vi "LcWebView_AlertDialog_Example2.vi"() -> ()   [LabVIEW 2018, in "LcWebView.lvclass"]
doc: "Inject javascript arguments"
uses:
  LcWebView.lvclass
  C:/Projects/LcWebView2/LcWebView/LcWebView_class/data/Microsoft.Web.WebView2.WinForms.dll
  data/Microsoft.Web.WebView2.WinForms.dll
panel:
  out "BrowserProcessId":u32
  out "Status Message":string
  in  "stop":bool
  in  "Web":refnum<k24>(container)
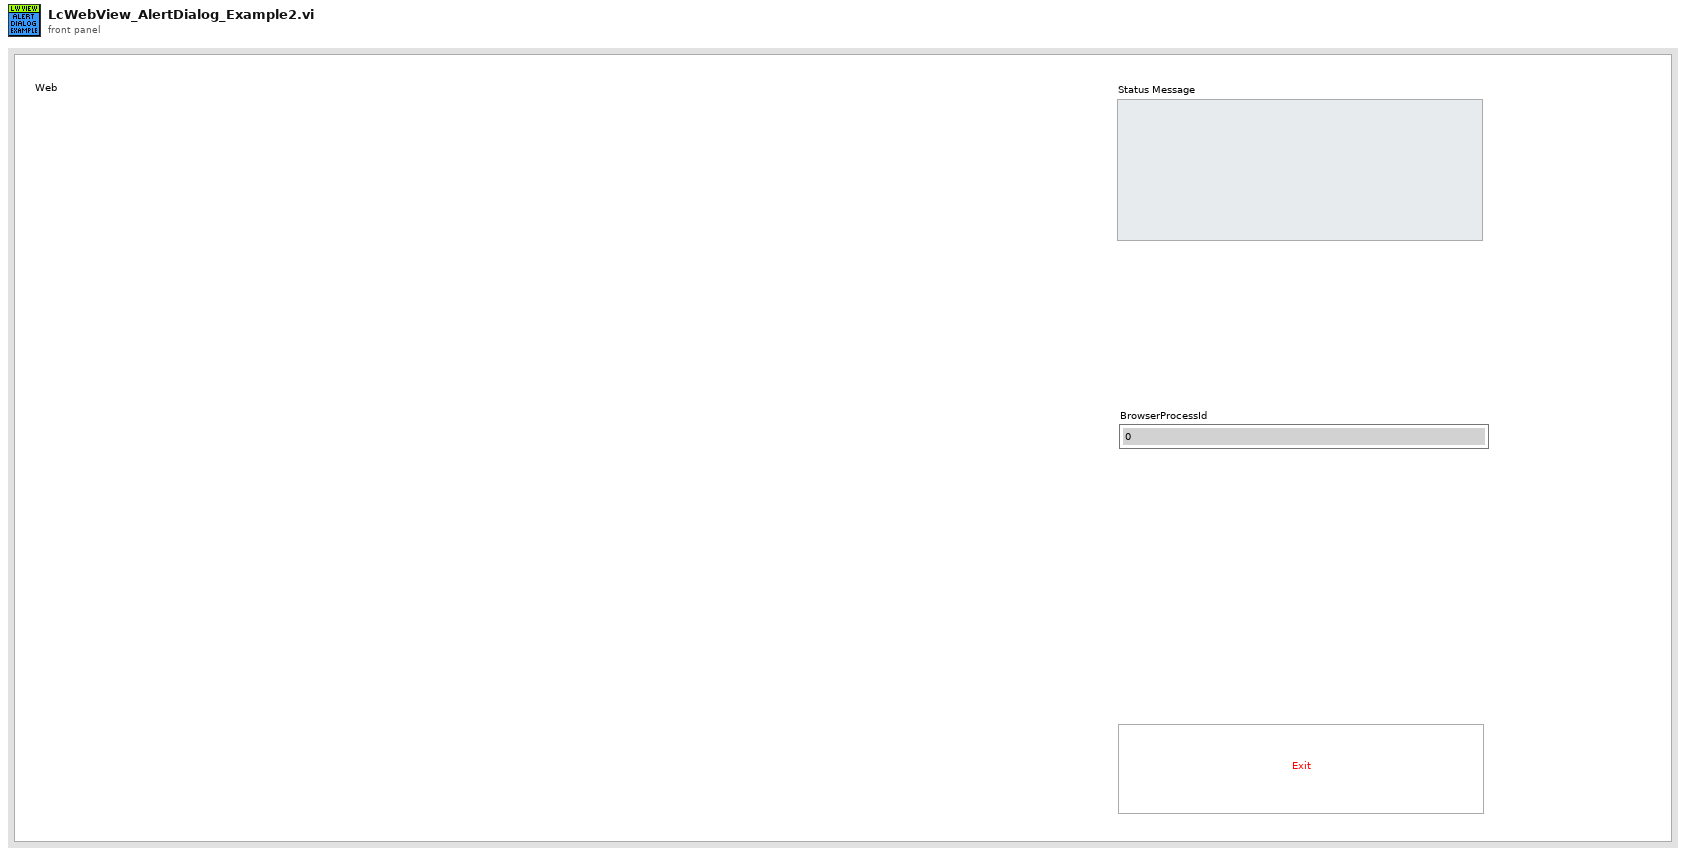
[diagram p1: front panel]
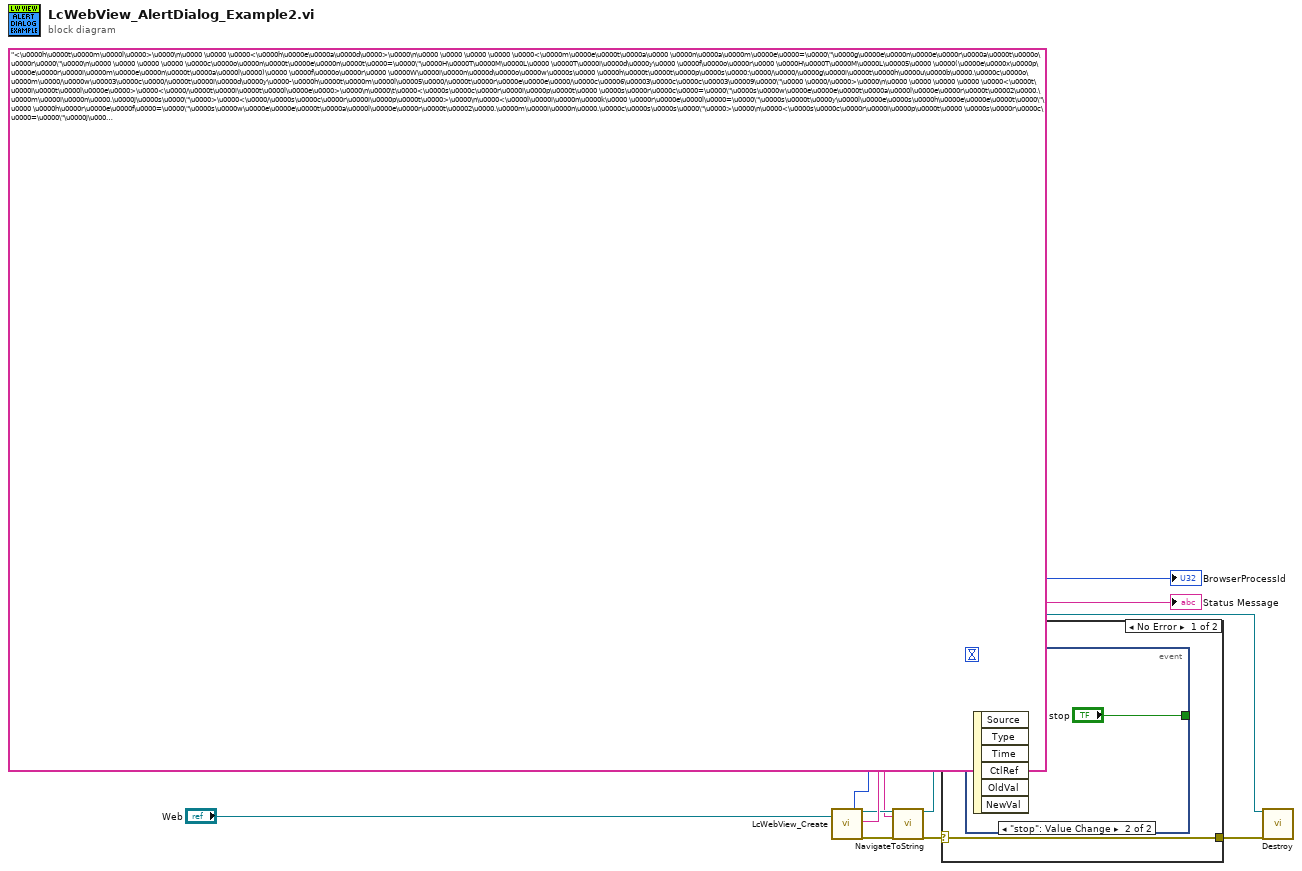
[diagram p0: block diagram]
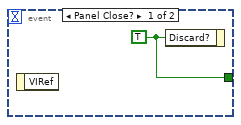
[diagram p2: hidden frame]
diagram:
  n1 = call "LcWebView_Create.vi"("Webview container"="Web") -> ("BrowserProcessId"=→"BrowserProcessId":u32, "reference out"=w6:refnum<class "LcWebView.lvclass">, "Status Message"=→"Status Message":string, "Error Out"=w5:errorcluster)  [unwired: 11 in, 4 out]
  n2 = call-dynamic "NavigateToString.vi"("reference in"=w6, "HTML Content"="<\u0000h\u0000t\u0000m\u0000l\u0000>\u0000\n\u0000 \u0000 \u0000<\u0000h\u0000e\u0000a\u0000d\u0000>\u0000\n\u0000 \u0000 \u0000 \u0000 \u0000<\u0000m\u0000e\u0000t\u0000a\u0000 \u0000n\u0000a\u0000m\u0000e\u0000=\u0000\"\u0000g\u0000e\u0000n\u0000e\u0000r\u0000a\u0000t\u0000o\u0000r\u0000\"\u0000\n\u0000 \u0000 \u0000 \u0000 \u0000c\u0000o\u0000n\u0000t\u0000e\u0000n\u0000t\u0000=\u0000\"\u0000H\u0000T\u0000M\u0000L\u0000 \u0000T\u0000i\u0000d\u0000y\u0000 \u0000f\u0000o\u0000r\u0000 \u0000H\u0000T\u0000M\u0000L\u00005\u0000 \u0000(\u0000e\u0000x\u0000p\u0000e\u0000r\u0000i\u0000m\u0000e\u0000n\u0000t\u0000a\u0000l\u0000)\u0000 \u0000f\u0000o\u0000r\u0000 \u0000W\u0000i\u0000n\u0000d\u0000o\u0000w\u0000s\u0000 \u0000h\u0000t\u0000t\u0000p\u0000s\u0000:\u0000/\u0000/\u0000g\u0000i\u0000t\u0000h\u0000u\u0000b\u0000.\u0000c\u0000o\u0000m\u0000/\u0000w\u00003\u0000c\u0000/\u0000t\u0000i\u0000d\u0000y\u0000-\u0000h\u0000t\u0000m\u0000l\u00005\u0000/\u0000t\u0000r\u0000e\u0000e\u0000/\u0000c\u00006\u00003\u0000c\u0000c\u00003\u00009\u0000\"\u0000 \u0000/\u0000>\u0000\n\u0000 \u0000 \u0000 \u0000 \u0000<\u0000t\u0000i\u0000t\u0000l\u0000e\u0000>\u0000<\u0000/\u0000t\u0000i\u0000t\u0000l\u0000e\u0000>\u0000\n\u0000\t\u0000<\u0000s\u0000c\u0000r\u0000i\u0000p\u0000t\u0000 \u0000s\u0000r\u0000c\u0000=\u0000\"\u0000s\u0000w\u0000e\u0000e\u0000t\u0000a\u0000l\u0000e\u0000r\u0000t\u00002\u0000.\u0000m\u0000i\u0000n\u0000.\u0000j\u0000s\u0000\"\u0000>\u0000<\u0000/\u0000s\u0000c\u0000r\u0000i\u0000p\u0000t\u0000>\u0000\n\u0000<\u0000l\u0000i\u0000n\u0000k\u0000 \u0000r\u0000e\u0000l\u0000=\u0000\"\u0000s\u0000t\u0000y\u0000l\u0000e\u0000s\u0000h\u0000e\u0000e\u0000t\u0000\"\u0000 \u0000h\u0000r\u0000e\u0000f\u0000=\u0000\"\u0000s\u0000w\u0000e\u0000e\u0000t\u0000a\u0000l\u0000e\u0000r\u0000t\u00002\u0000.\u0000m\u0000i\u0000n\u0000.\u0000c\u0000s\u0000s\u0000\"\u0000>\u0000\n\u0000<\u0000s\u0000c\u0000r\u0000i\u0000p\u0000t\u0000 \u0000s\u0000r\u0000c\u0000=\u0000\"\u0000j\u0000a\u0000v\u0000a\u0000s\u0000c\u0000r\u0000i\u0000p\u0000t\u0000.\u0000j\u0000s\u0000\"\u0000>\u0000\n\u0000f\u0000u\u0000...", "Error In"=w5) -> ("reference out"=w3:refnum<class "LcWebView.lvclass">, "Error Out"=w2:errorcluster)  [unwired: 14 in, 1 out]
  n3 = case shown="No Error" w2 {
    selector: w2 -> [w10 w13]
    tunnel: [w10 w13] -> w1
    frame No Error {
      n4 = event shown="[1] \"stop\": Value Change" {
        selector: _ -> [_ _]
        dyn-events: _ -> [_ _]
        timeout: _ -> [_ _]
        tunnel: [w11 "stop"] -> _
        event Panel Close? {
          w11 = TRUE ("Discard?")
          n5 = event-data() -> ()  [unwired: 1 in, 1 out]
          n6 = event-data("Discard?"=w11) -> ()  [unwired: 1 in, 1 out]
        }
        event "stop": Value Change {
          n7 = event-data() -> ()  [unwired: 1 in, 6 out]
        }
      }
    }
    frame Error {
    }
  }
  n8 = call-dynamic "Destroy.vi"("reference in"=w3, "Error In"=w1) -> ()  [unwired: 16 in, 2 out]
